vi "Problemas monitoreo 2.vi"() -> ()   [LabVIEW 2020]
uses:
  <vilib>/Instr/_visa.llb/VISA Configure Serial Port (Instr).vi
panel:
  out "concatenated string 2":string
  in  "string":string
  in  "Boolean 2":bool
  in  "Boolean":bool
  out "concatenated string":string
  in  "VISA resource name":refnum<visa-resource-name>
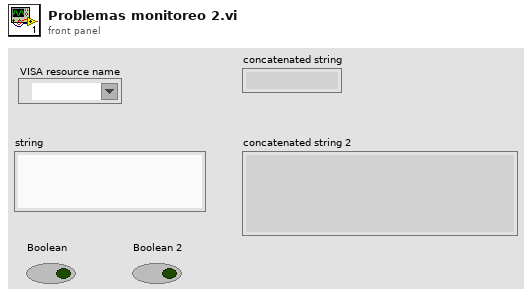
[diagram p1: front panel]
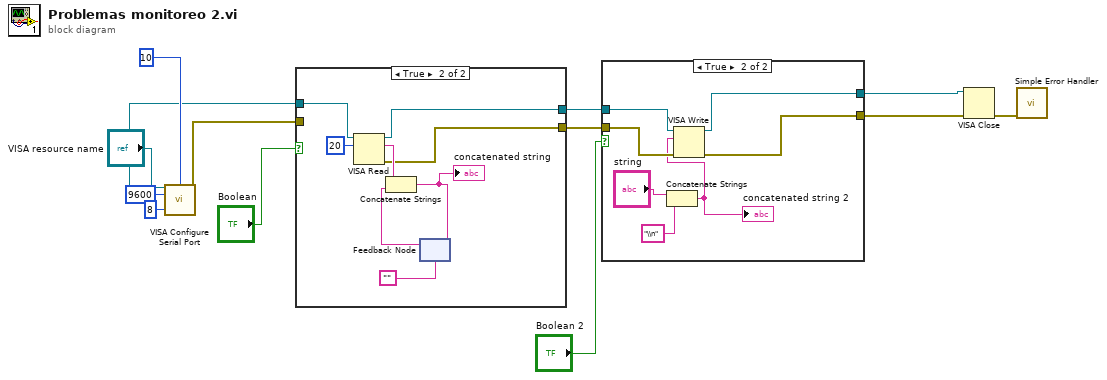
[diagram p0: block diagram]
diagram:
  n1 = call-poly "VISA Configure Serial Port"("VISA resource name"="VISA resource name", "termination char\n(0xA = '\\n' = LF)"=u8 10 ("termination char\n(0xA = '\\n' = LF)"), "baud rate (9600)"=u32 9600, "data bits (8)"=u16 8) -> ("VISA resource name out"=w4:refnum<visa-resource-name>, "error out"=w3:errorcluster)  [unwired: 10 in]
  n2 = case shown="True" "Boolean" {
    tunnel: w4 -> [w15 w21]
    tunnel: [w15 w20] -> w5
    tunnel: w3 -> [w14 _]
    tunnel: [w14 w19] -> w7
    frame False {
    }
    frame True {
      n3 = VISA Read(VISA resource name=w21, byte count=u32 20) -> (VISA resource name out=w20:refnum<visa-resource-name>, read buffer=w22:string, error out=w19:errorcluster)  [unwired: 1 in, 1 out]
      n4 = feedback #1("") -> (w17:string)
      n5 = Concatenate Strings(w22, w17) -> (w18:string)
      "concatenated string" <- w18
      n6 = feedback-in #1(w18) -> ()
    }
  }
  n7 = case shown="True" "Boolean 2" {
    tunnel: w5 -> [w24 w31]
    tunnel: w7 -> [w25 w29]
    tunnel: [w24 w32] -> w2
    tunnel: [w25 w30] -> w1
    frame False {
    }
    frame True {
      n8 = Concatenate Strings("string", "\\n" ("string")) -> (w28:string)
      "concatenated string 2" <- w28
      n9 = VISA Write(VISA resource name=w31, write buffer=w28, error in (no error)=w29) -> (VISA resource name out=w32:refnum<visa-resource-name>, error out=w30:errorcluster)  [unwired: 1 out]
    }
  }
  n10 = VISA Close(VISA resource name=w2, error in (no error)=w1) -> (error out=w10:errorcluster)
  n11 = call <vilib>:"Simple Error Handler.vi"("error in (no error)"=w10) -> ()  [unwired: 4 in, 5 out]
